vi "Write Log Level.vi"(8 "error in (no error)":errorcluster, 10 "Log Level":T1, 11 "Logger in":refnum<class "Generic Logger.lvclass">) -> (0 "error out":errorcluster, 3 "Logger out":refnum<class "Generic Logger.lvclass">)   [LabVIEW 2020, in "Logging.lvlib" / "Generic Logger.lvclass"]
uses:
  Generic Logger.lvclass
  Define/Log Level.ctl
  Generic Logger.lvclass/Generic Logger.ctl
  Logging.lvlib
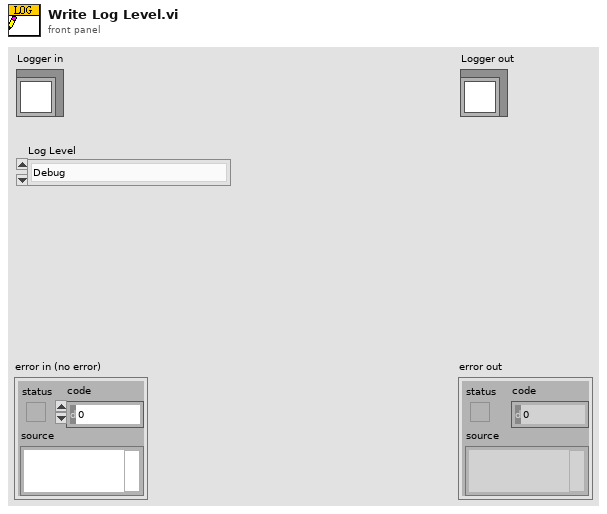
[diagram p1: front panel]
types:
  T1 = typedef "Logging.lvlib/Log Level.ctl" = enum16{"Debug", "Info", "Warn", "Error"}
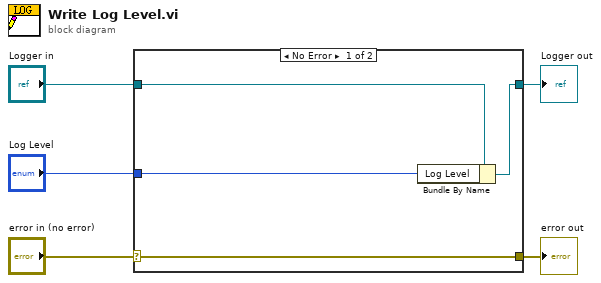
[diagram p0: block diagram]
diagram:
  n1 = case shown="No Error" "error in (no error)" {
    selector: "error in (no error)" -> [w9 w10]
    tunnel: [w9 w10] -> w4
    tunnel: [w7 w11] -> w2
    tunnel: "Logger in" -> [w8 w11]
    tunnel: "Log Level" -> [w6 _]
    frame No Error {
      n2 = Bundle By Name(cluster=w8, "Log Level"=w6) -> (w7:refnum<class "Generic Logger.lvclass">)
    }
    frame Error {
    }
  }
  "error out" <- w4
  "Logger out" <- w2
